vi "DQMH Scripting Tools Panel.vi"() -> ()   [LabVIEW 2019, in "Panther Dashboard.lvlib"]
uses:
  Panther Dashboard.lvlib
  DQMH Tools Menu--enum.ctl
panel:
  in  "About":bool=TRUE
  in  "Add Event":bool caption="Add\nEvent"
  in  "Remove Event":bool caption="Remove\nEvent"
  in  "Convert Event":bool caption="Convert\nEvent"
  in  "Rename Event":bool caption="Rename\nEvent"
  in  "Add Module":bool caption="Add\nModule"
  in  "Rename Module":bool caption="Rename\nModule"
  in  "Validate Module":bool caption="Validate\nModule"
  in  "Create Module Template":bool caption="Create\nTemplate"
  in  "Add Unit Test":bool caption="Add \nUnit Test"
  in  "Create RT Tester":bool caption="Create RT\nTester"
  in  "Theme":bool=TRUE
  in  "Generate Antidoc":bool caption="Generate\nAntidoc"
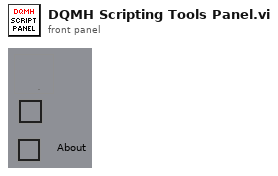
[diagram p1: front panel]
types:
  T1 = typedef "Panther Dashboard.lvlib/Broadcast Events--cluster.ctl" = cluster{"Module Did Init":refnum<user-event>, "Status Updated":refnum<user-event>, "Error Reported":refnum<user-event>, "Module Did Stop":refnum<user-event>, "Update Module Execution Status":refnum<user-event>, "References Updated":refnum<user-event>, "Projects Updated":refnum<user-event>, "Targets Updated":refnum<user-event>}
  T2 = typedef "Panther Dashboard.lvlib/DQMH Tools Menu--enum.ctl" = enum16{"Create New DQMH Event", "Remove DQMH Event", "Convert DQMH Event", "Rename DQMH Event", "Add New DQMH Module", "Create RT Tester", "Rename DQMH Module", "Validate DQMH Module", "Create DQMH Module Template", "New DQMH  Unit Test"}
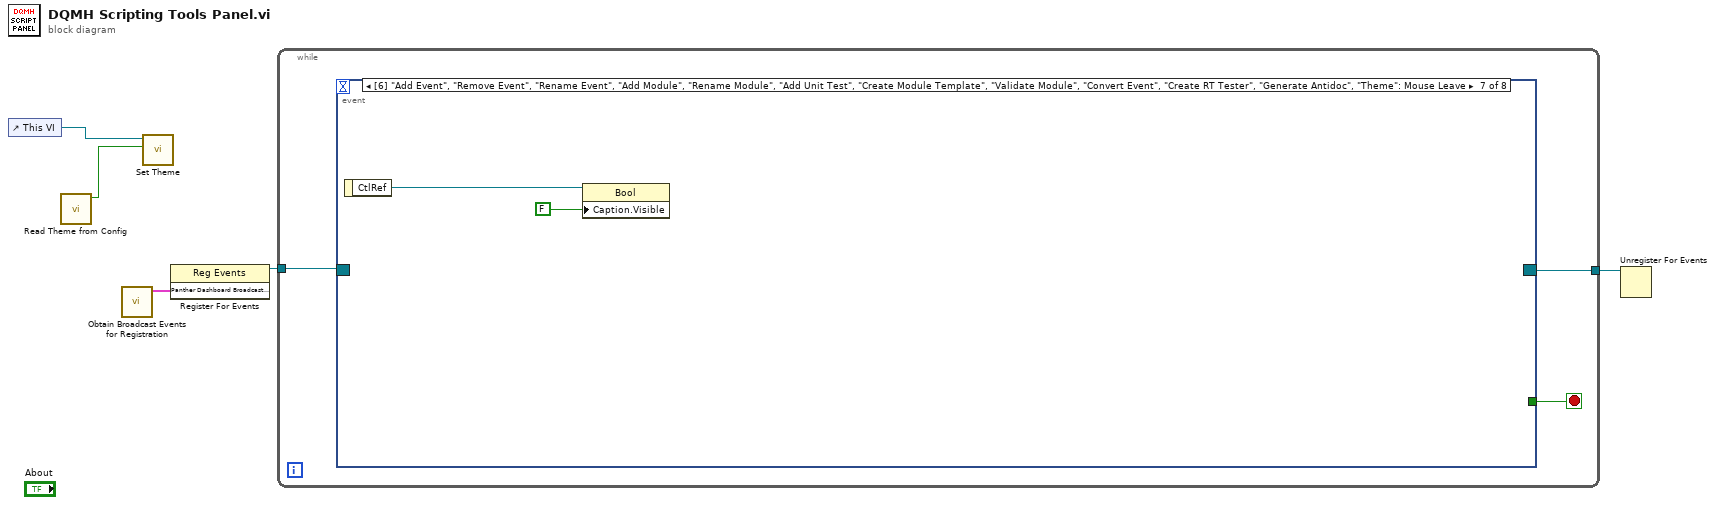
[diagram p0: block diagram]
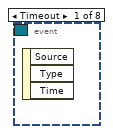
[diagram p2: hidden frame]
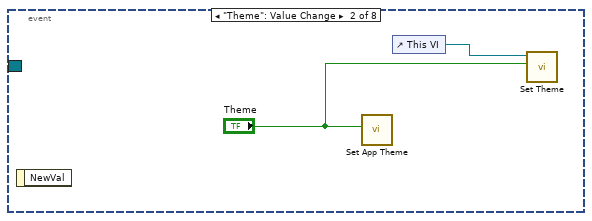
[diagram p3: hidden frame]
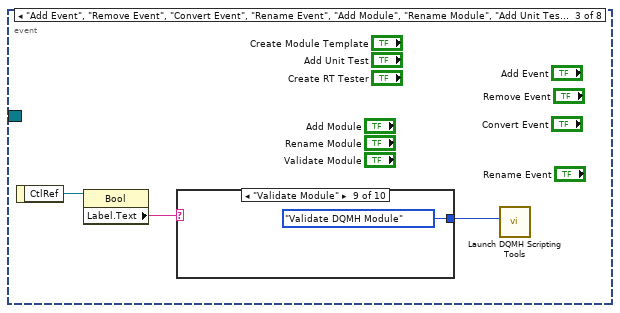
[diagram p4: hidden frame]
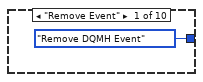
[diagram p5: hidden frame]
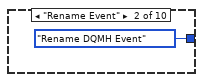
[diagram p6: hidden frame]
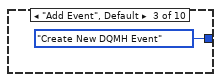
[diagram p7: hidden frame]
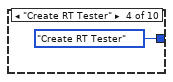
[diagram p8: hidden frame]
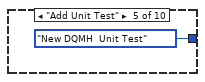
[diagram p9: hidden frame]
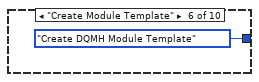
[diagram p10: hidden frame]
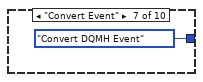
[diagram p11: hidden frame]
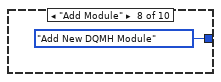
[diagram p12: hidden frame]
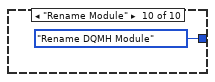
[diagram p13: hidden frame]
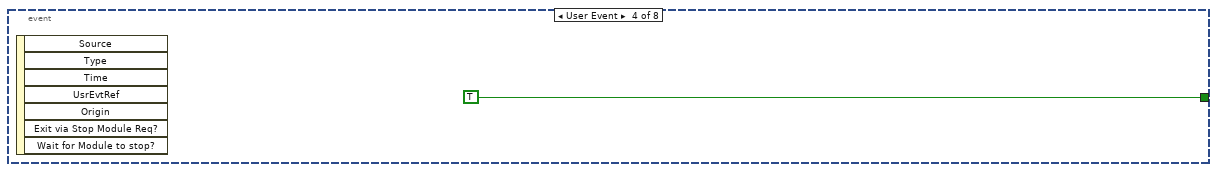
[diagram p14: hidden frame]
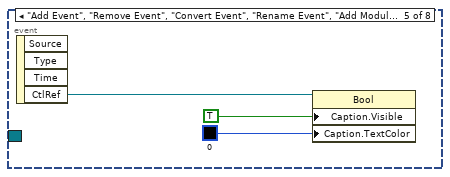
[diagram p15: hidden frame]
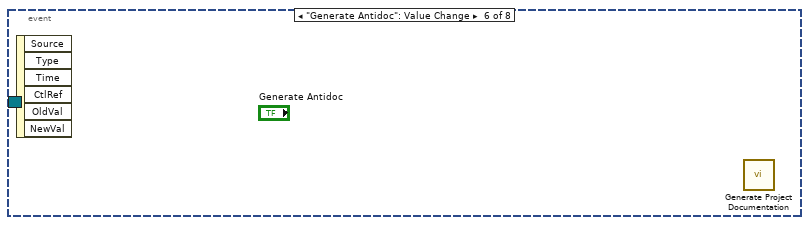
[diagram p16: hidden frame]
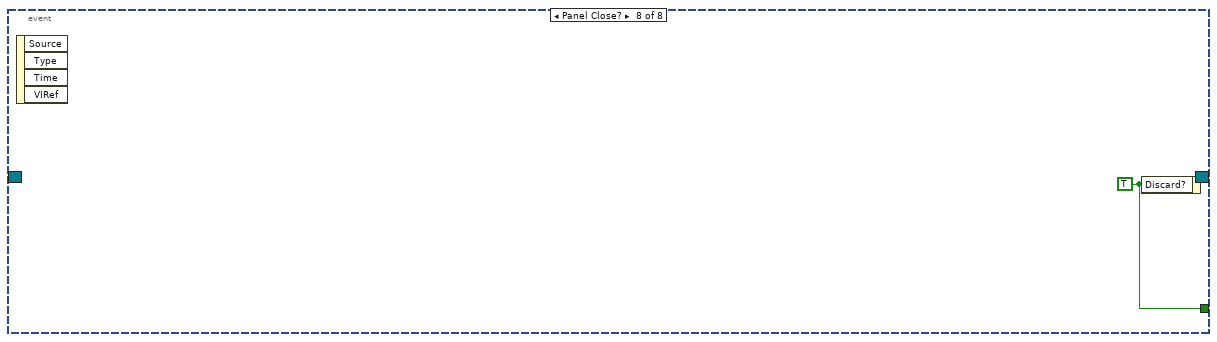
[diagram p17: hidden frame]
diagram:
  n1 = control-ref of="This VI"() -> (w2:refnum<vi>)
  n2 = call "Read Theme from Config.vi"() -> ("Theme"=w1:bool)  [unwired: 10 in, 1 out]
  n3 = call "Obtain Broadcast Events for Registration.vi"() -> ("Panther Dashboard Broadcast Events"=w4:T1)  [unwired: 9 in, 2 out]
  n4 = call "Set Theme.vi"("Dark?"=w1, "VI in"=w2) -> ()  [unwired: 10 in]
  n5 = register-events(w4) -> (reference out=w5:refnum<event-registration>)  [unwired: 2 in, 1 out]
  n6 = while {
    tunnel: w5 -> [w8]
    tunnel: [w6] -> w3
    stop <- w7 stop-if-true
    n7 = event shown="[6] \"Add Event\", \"Remove Event\", \"Rename Event\", \"Add Module\", \"Rename Module\", \"Add Unit Test\", \"Create Module Template\", \"Validate Module\", \"Convert Event\", \"Create RT Tester\", \"Generate Antidoc\", \"Theme\": Mouse Leave" {
      selector: w8 -> [_ _ _ _ _ _ _ _]
      dyn-events: [_ _ _ _ _ _ _ _] -> w6
      timeout: _ -> [_ _ _ _ _ _ _ _]
      tunnel: [_ _ _ TRUE _ _ _ w30] -> w7
      event Timeout {
        n8 = event-data() -> ()  [unwired: 1 in, 3 out]
      }
      event "Theme": Value Change {
        n9 = event-data() -> ()  [unwired: 1 in, 1 out]
        n10 = call "Set App Theme.vi"("Theme"="Theme") -> ()  [unwired: 10 in, 1 out]
        n11 = control-ref of="This VI"() -> (w10:refnum<vi>)
        n12 = call "Set Theme.vi"("Dark?"="Theme", "VI in"=w10) -> ()  [unwired: 10 in]
      }
      event "Add Event", "Remove Event", "Convert Event", "Rename Event", "Add Module", "Rename Module", "Add Unit Test", "Create Module Template", "Validate Module", "Create RT Tester": Value Change {
        n13 = event-data() -> ("CtlRef"=w13:refnum<vi>)  [unwired: 1 in]
        n14 = property class="Bool"(reference=w13) -> ("Label.Text"=w12:string)  [unwired: 1 in, 2 out]
        n15 = case shown="\"Validate Module\"" w12 {
          tunnel: [DQMH_Tools_Menu--enum."Remove DQMH Event" ("DQMH Tools") DQMH_Tools_Menu--enum."Rename DQMH Event" ("DQMH Tools") DQMH_Tools_Menu--enum."Create New DQMH Event" ("DQMH Tools") DQMH_Tools_Menu--enum."Create RT Tester" ("DQMH Tools") DQMH_Tools_Menu--enum."New DQMH  Unit Test" ("DQMH Tools") DQMH_Tools_Menu--enum."Create DQMH Module Template" ("DQMH Tools") DQMH_Tools_Menu--enum."Convert DQMH Event" ("DQMH Tools") DQMH_Tools_Menu--enum."Add New DQMH Module" ("DQMH Tools") DQMH_Tools_Menu--enum."Validate DQMH Module" ("DQMH Tools") DQMH_Tools_Menu--enum."Rename DQMH Module" ("DQMH Tools")] -> w11
          frame "Remove Event" {
          }
          frame "Rename Event" {
          }
          frame "Add Event", Default {
          }
          frame "Create RT Tester" {
          }
          frame "Add Unit Test" {
          }
          frame "Create Module Template" {
          }
          frame "Convert Event" {
          }
          frame "Add Module" {
          }
          frame "Validate Module" {
          }
          frame "Rename Module" {
          }
        }
        n16 = call "Launch DQMH Scripting Tools.vi"("Scripting Tool"=w11) -> ()  [unwired: 10 in, 1 out]
      }
      event User Event {
        n17 = event-data() -> ()  [unwired: 1 in, 7 out]
      }
      event "Add Event", "Remove Event", "Convert Event", "Rename Event", "Add Module", "Rename Module", "Add Unit Test", "Create Module Template", "Validate Module", "Create RT Tester", "Generate Antidoc", "Theme": Mouse Enter {
        n18 = event-data() -> ("CtlRef"=w27:refnum<vi>)  [unwired: 1 in, 3 out]
        n19 = property class="Bool"(reference=w27, "Caption.Visible"=TRUE, "Caption.TextColor"=u32 0) -> ()  [unwired: 1 in, 2 out]
      }
      event "Generate Antidoc": Value Change {
        n20 = event-data() -> ()  [unwired: 1 in, 6 out]
        n21 = call "Generate Project Documentation.vi"() -> ()  [unwired: 11 in, 1 out]
      }
      event "Add Event", "Remove Event", "Rename Event", "Add Module", "Rename Module", "Add Unit Test", "Create Module Template", "Validate Module", "Convert Event", "Create RT Tester", "Generate Antidoc", "Theme": Mouse Leave {
        n22 = event-data() -> ("CtlRef"=w29:refnum<vi>)  [unwired: 1 in]
        n23 = property class="Bool"(reference=w29, "Caption.Visible"=FALSE) -> ()  [unwired: 1 in, 2 out]
      }
      event Panel Close? {
        w30 = TRUE ("Discard?")
        n24 = event-data() -> ()  [unwired: 1 in, 4 out]
        n25 = event-data("Discard?"=w30) -> ()  [unwired: 1 in, 1 out]
      }
    }
  }
  n26 = Unregister For Events(event registration refnum=w3) -> ()  [unwired: 1 in, 1 out]
